vi "HXG2_DitheringAdder.vi"() -> (3 "-.2 to .2 (mA)":dbl format="%#_3f")   [LabVIEW 2012]
panel:
  out "mA":dbl format="%#.8f"
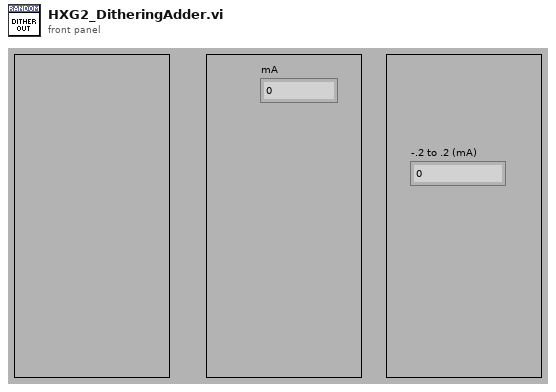
[diagram p1: front panel]
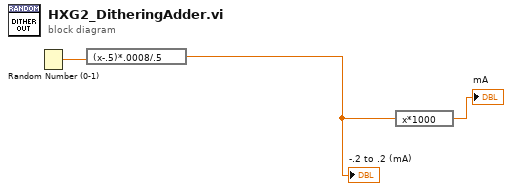
[diagram p0: block diagram]
diagram:
  n1 = Random Number (0-1)() -> (number: 0 to 1=w3:dbl)
  n2 = expression code="(x-.5)*.0008/.5"(w3) -> (w2:dbl)
  "-.2 to .2 (mA)" <- w2
  n3 = expression code="x*1000"(w2) -> (→"mA":dbl)
